vi "rsscope_FormatSearchNameTBTOWordInt32_ReadCallback.vi"(5 "Attribute":T1={"Identifier"="", "Descriptive Name"="", "Data Type"=enum."Integer 32", "Command"="", "Access"=enum."Read/Write", "Range Table"="", "Read Callback"="", "Write Callback"="", "Supported Models"="", "Instrument Options"="", "Index"=0, "OPC Wait"=FALSE, "No Status Check"=FALSE, "Cache Only"=FALSE}, 7 "Repeated Capability":string, 8 "error in (no error)":errorcluster, 11 "VISA resource name":refnum<visa-resource-name>) -> (0 "error out":errorcluster, 2 "Attribute Value I32":i32, 3 "VISA resource name out":refnum<visa-resource-name>)   [LabVIEW 2014]
doc: "This VI sets the attribute value.\n\nThis is a low-level VI that you can use to set the values of instrument-specific properties and inherent IVI properties. If the property represents an instrument state, this VI performs instrument I/O in the following cases:\n\n- State caching is disabled for the entire session or for the particular property.\n\n- State caching is enabled and the currently cached value is invalid or is different than the value you specify. \n\nThis instrument driver contains high-level VIs that set most of the instrument properties. It is best to use the high-level driver VIs as much as possible. They handle order dependencies and multithread locking for you. In addition, they perform status checking only after setting all of the properties. In contrast, when you set multiple properties using the SetAttribute VIs, the VIs check the instrument status after each call.\n\nAlso, when state caching is enabled, the high-level VIs that configure multiple properties perform instrument I/O only for the properties whose value you change. Thus, you can safely call the high-level VIs without the penalty of redundant instrument I/O."
uses:
  rsidr_core.llb/rsscope_rsidr_core.lvlib
  rsidr_core.llb/type_Attribute_Data_Type.ctl
  rsidr_core.llb/type_Attribute.ctl
  rsidr_core.llb/type_ReadWriteAccess.ctl
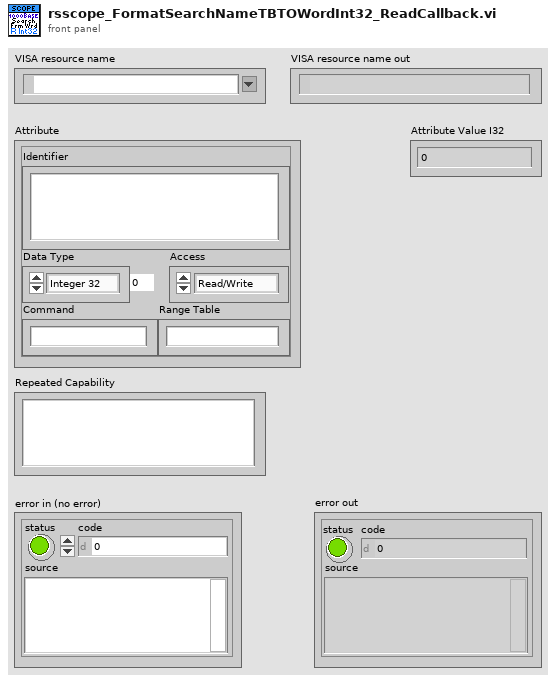
[diagram p1: front panel]
types:
  T1 = typedef "rsscope_rsidr_core.lvlib/type_Attribute.ctl" = cluster{"Identifier":string, "Descriptive Name":string, "Data Type":T2, "Command":string, "Access":T3, "Range Table":string, "Read Callback":string, "Write Callback":string, "Supported Models":string, "Instrument Options":string, "Index":i32, "OPC Wait":bool, "No Status Check":bool, "Cache Only":bool}
  T2 = typedef "rsscope_rsidr_core.lvlib/type_Attribute_Data_Type.ctl" = enum16{"Integer 32", "Double", "String", "Boolean", "None", "Integer 64", "RawString"}
  T3 = typedef "rsscope_rsidr_core.lvlib/type_ReadWriteAccess.ctl" = enum16{"Read Only", "Write Only", "Read/Write"}
  T4 = typedef "rsscope_rsidr_core.lvlib/type_Session_Data.ctl" = cluster{"IDN string":string, "Instrument FW":string, "Instr type":string, "Instr type for err. msg.":string, "Installed Options":string[], "Ignore Error Messages":string, "Logging params":variant, "OPC Timeout":i32, "VISA Timeout":i32, "STB Poll VISA Timeout":i32, "Additional Flags":i32, "Wait Before Read":i32, "Wait Before Write":i32, "Option String Flags":i32, "IO Segment Size":i64, "VISA Access Mode":T5, "Interface Type":T6, "OPC Wait Mode":T7, "Bin Float Number  Format":T8, "Bin Integer Number Format":T9, "Simulate":bool, "VXIcapable":bool, "Duplicate Session":bool, "Add LF to Write":bool, "Logging":bool, "Fast Sweep":bool, "Query Instrument Status":bool, "Check Range":bool, "Check Options":bool}
  T5 = typedef "rsscope_rsidr_core.lvlib/type_VisaAccessMode.ctl" = u16
  T6 = typedef "rsscope_rsidr_core.lvlib/type_InterfaceType.ctl" = enum16{"Unknown", "GPIB", "VXI", "GPIB_VXI", "ASRL", "PXI", "TCPIP", "USB", "SOCKET"}
  T7 = typedef "rsscope_rsidr_core.lvlib/type_OPC_Wait_Mode.ctl" = enum16{"STBpolling", "STBpollingSlow", "STBpollingSuperSlow", "ServiceRequest", "OPCquery"}
  T8 = typedef "rsscope_rsidr_core.lvlib/type_Binary_Float_Number_Format.ctl" = enum16{"Float_4_Bytes_Swapped", "Float_4_Bytes", "Double_8_Bytes_Swapped", "Double_8_Bytes"}
  T9 = typedef "rsscope_rsidr_core.lvlib/type_Binary_Integer_Number_Format.ctl" = enum16{"Int32_4_Bytes_Swapped", "Int32_4 Bytes", "Int16_2_Bytes_Swapped", "Int16_2_Bytes"}
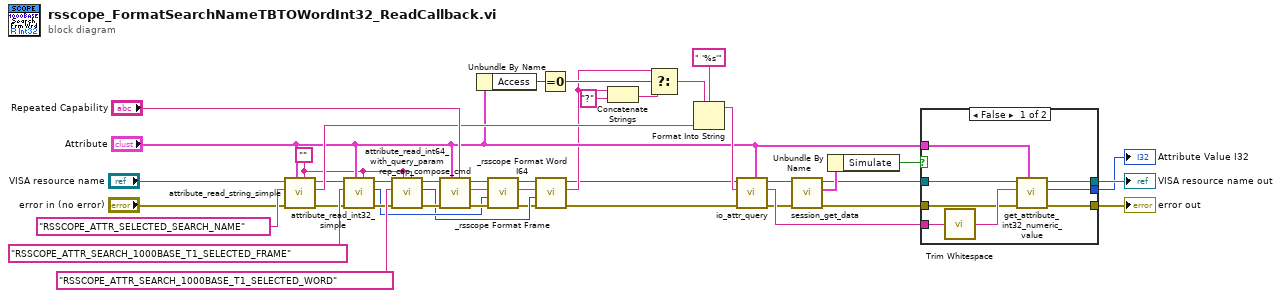
[diagram p0: block diagram]
diagram:
  w1 = "" ("Empty String Constant")
  n1 = call "attribute_read_string_simple.vi"("Repeated Capability"=w1, "Attribute"="Attribute", "error in"="error in (no error)", "Direct Attribute ID (\"\")"="RSSCOPE_ATTR_SELECTED_SEARCH_NAME" ("Direct Attribute ID (\"\")"), "VISA resource name"="VISA resource name") -> ("error out"=w19:errorcluster, "String out"=w38:string, "VISA resource name out"=w20:refnum<visa-resource-name>)  [unwired: 4 in]
  n2 = call "attribute_read_int32_simple.vi"("Repeated Capability"=w1, "Attribute"="Attribute", "error in"=w19, "Direct Attribute ID (\"\")"="RSSCOPE_ATTR_SEARCH_1000BASE_T1_SELECTED_FRAME" ("Direct Attribute ID (\"\")"), "VISA resource name"=w20) -> ("error out"=w16:errorcluster, "Int32 out"=w9:i32, "VISA resource name out"=w17:refnum<visa-resource-name>)  [unwired: 4 in]
  n3 = call "attribute_read_int64_with_query_param.vi"("Query Parameter (None)"=w1, "Repeated Capability"=w1, "error in"=w16, "Attribute ID"="RSSCOPE_ATTR_SEARCH_1000BASE_T1_SELECTED_WORD" ("Direct Attribute ID (\"\")"), "VISA resource name"=w17) -> ("error out"=w13:errorcluster, "Int64 out"=w6:i64, "VISA resource name out"=w14:refnum<visa-resource-name>)  [unwired: 4 in]
  n4 = call "rep_cap_compose_cmd.vi"("Repeated Capability"="Repeated Capability", "Attribute"="Attribute", "error in"=w13, "VISA resource name"=w14) -> ("error out"=w10:errorcluster, "Command out"=w12:string, "VISA resource name out"=w11:refnum<visa-resource-name>)  [unwired: 5 in]
  n5 = Unbundle By Name("Attribute") -> ("Access"=w34:T3)
  n6 = call "_rsscope Format Frame.vi"("error in (no error)"=w10, "Frame (1)"=w9, "Input String"=w12, "VISA resource name"=w11) -> ("error out"=w5:errorcluster, "Output String"=w8:string, "VISA resource name out"=w7:refnum<visa-resource-name>)  [unwired: 5 in]
  n7 = call "_rsscope Format Word I64.vi"("error in (no error)"=w5, "Word (1)"=w6, "Input String"=w8, "VISA resource name"=w7) -> ("error out"=w2:errorcluster, "Output String"=w4:string, "VISA resource name out"=w3:refnum<visa-resource-name>)  [unwired: 5 in]
  n8 = Equal To 0?(x=w34) -> (x = 0?=w33:bool)
  n9 = Concatenate Strings(w4, "?" ("string")) -> (w36:string)
  n10 = Select(t=w4, s=w33, f=w36) -> (s? t:f=w32:string)
  n11 = Format Into String(format string=" '%s'", initial string=w32, w38) -> (resulting string=w37:string)  [unwired: 1 in, 1 out]
  n12 = call "io_attr_query.vi"("Attribute"="Attribute", "error in"=w2, "write buffer"=w37, "VISA resource name"=w3) -> ("error out"=w23:errorcluster, "read buffer"=w24:string, "VISA resource name out"=w22:refnum<visa-resource-name>)  [unwired: 5 in]
  n13 = call "session_get_data.vi"("error in"=w23, "VISA resource name"=w22) -> ("error out"=w30:errorcluster, "Session User Data out"=w31:T4, "VISA resource name out"=w29:refnum<visa-resource-name>)  [unwired: 6 in, 1 out]
  n14 = Unbundle By Name(w31) -> ("Simulate"=w28:bool)
  n15 = case shown="False" w28 {
    tunnel: [w48 w53] -> w26
    tunnel: [w47 w52] -> w27
    tunnel: [w50 _] -> w25
    tunnel: "Attribute" -> [w49 _]
    tunnel: w30 -> [w45 w53]
    tunnel: w29 -> [w44 w52]
    tunnel: w24 -> [w46 _]
    frame False {
      n16 = call <vilib>:"Trim Whitespace.vi"("string"=w46) -> ("trimmed string"=w51:string)  [unwired: 1 in]
      n17 = call "get_attribute_int32_numeric_value.vi"("Attribute"=w49, "error in"=w45, "Cmd Value in"=w51, "VISA resource name"=w44) -> ("error out"=w48:errorcluster, "Int32 value out"=w50:i32, "VISA resource name out"=w47:refnum<visa-resource-name>)  [unwired: 5 in]
    }
    frame True {
    }
  }
  "error out" <- w26
  "VISA resource name out" <- w27
  "Attribute Value I32" <- w25
